vi "CapacityTest.vi"() -> ()   [LabVIEW 2020]
uses:
  <instrlib>/NH Research Regenerative Test Series/Public/Configure/Output Safety.ctl
  <vilib>/DAQmx/read.llb/DAQmx Read (Analog 1D DBL NChan 1Samp).vi
  <vilib>/DAQmx/miscellaneous.llb/DAQmx Fill In Error Info.vi
  <instrlib>/NH Research Regenerative Test Series/Public/Data/Read (Ave Current).vi
  <instrlib>/NH Research Regenerative Test Series/Public/Data/Low Level/Fetch (Ave Voltage).vi
  <instrlib>/NH Research Regenerative Test Series/Public/Data/Low Level/Fetch (Ave True Power).vi
  <instrlib>/NH Research Regenerative Test Series/NH Research Regenerative Test Series.lvlib
panel:
  out "ChamberTemp":dbl
  out "BatteryTemp":dbl
  out "Task error out":errorcluster
  out "String":string
  in  "Output Safety":T1
  out "Filename Out":path
  in  "DAQmx Task Name":refnum<k21>
  out "Voltage Compare":dbl
  in  "Path":path
  in  "Discharge Voltage Setpoint (0 V)":dbl
  out "Ave Current (A)":dbl
  out "Ave Voltage (V)":dbl
  out "Ave True Power (W)":dbl
  out "Status Byte Register":T2
  in  "Logical Instrument Number":u32=1
  in  "Current Setpoint (0 A)":dbl format="%#.6g"
  in  "Voltage Setpoint (0 V)":dbl format="%#.6g"
  in  "Battery Detect Voltage (0V)":dbl format="%#.6g"
  in  "VISA resource name":refnum<visa-resource-name>
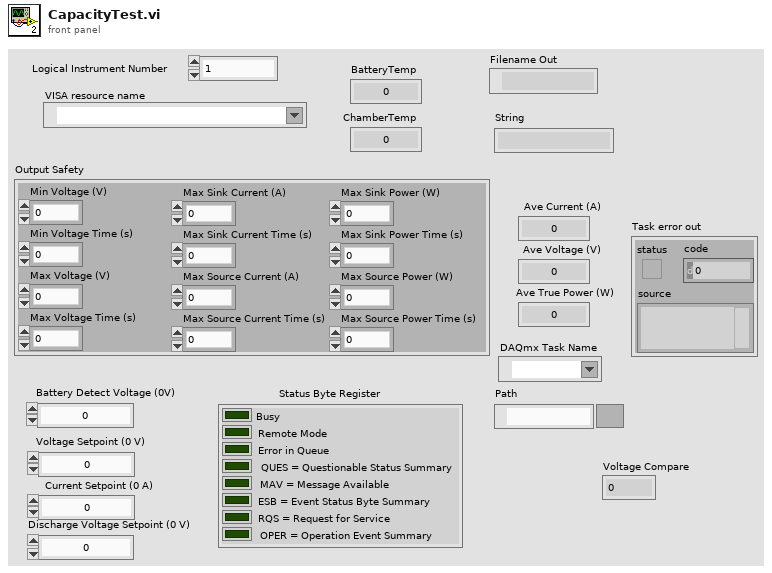
[diagram p1: front panel]
types:
  T1 = typedef "NH Research Regenerative Test Series.lvlib/Output Safety.ctl" = cluster{"Min Voltage (V)":dbl, "Min Voltage Time (s)":dbl, "Max Voltage (V)":dbl, "Max Voltage Time (s)":dbl, "Max Sink Current (A)":dbl, "Max Sink Current Time (s)":dbl, "Max Source Current (A)":dbl, "Max Source Current Time (s)":dbl, "Max Sink Power (W)":dbl, "Max Sink Power Time (s)":dbl, "Max Source Power (W)":dbl, "Max Source Power Time (s)":dbl}
  T2 = cluster{"Busy":bool, "Remote Mode":bool, "Error in Queue":bool, "QUES = Questionable Status Summary":bool, "MAV = Message Available":bool, "ESB = Event Status Byte Summary":bool, "RQS = Request for Service":bool, "OPER = Operation Event Summary":bool}
  T3 = cluster{"data[0]":dbl, "data[1]":dbl, "data[2]":dbl, "data[3]":dbl, "data[4]":dbl, "data[5]":dbl, "data[6]":dbl, "data[7]":dbl, "data[8]":dbl}
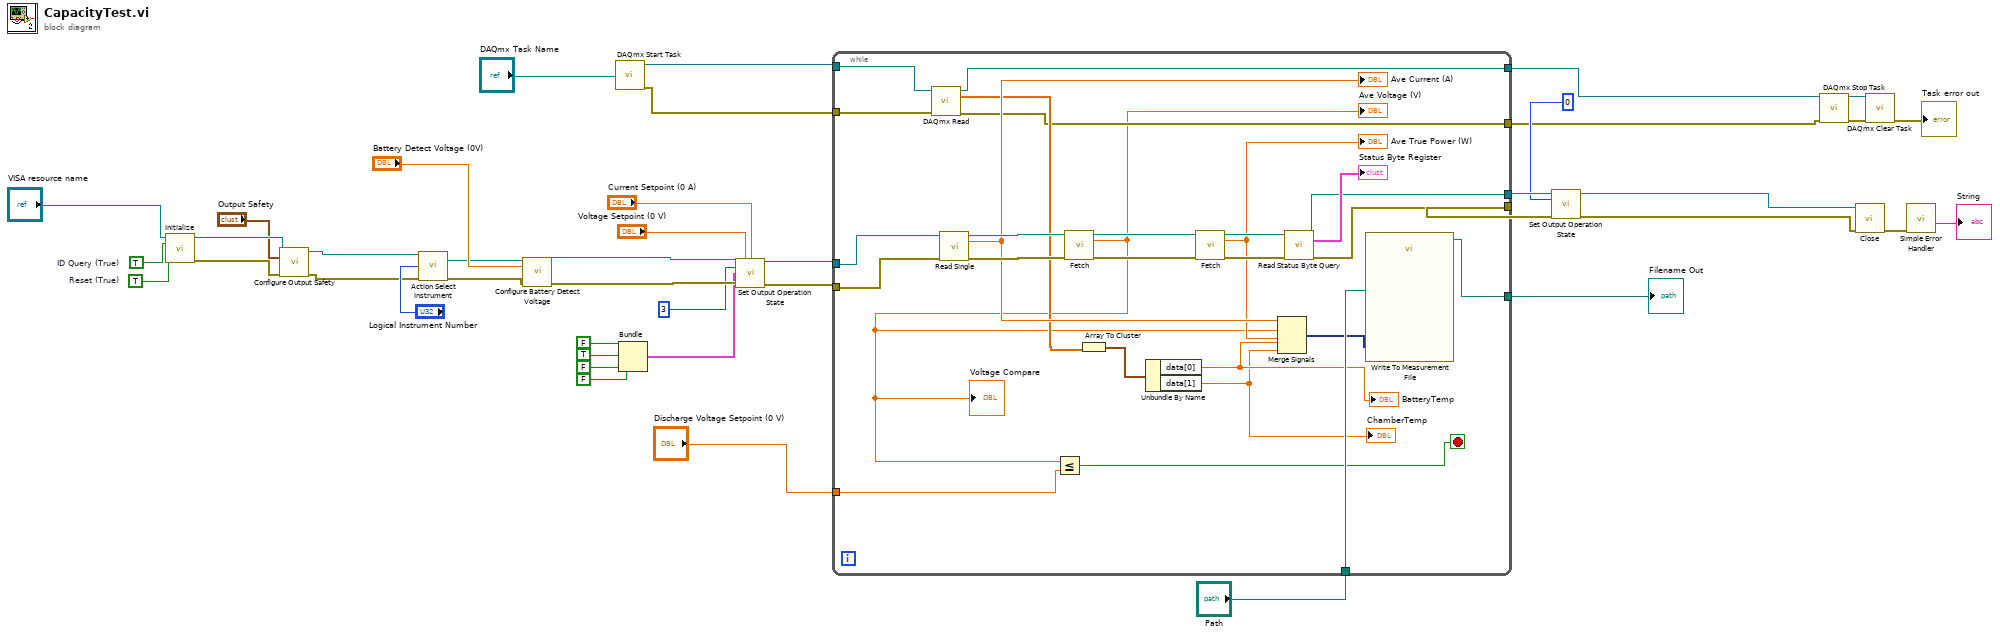
[diagram p0: block diagram]
diagram:
  w20 = TRUE  # ID Query (True)
  w19 = TRUE  # Reset (True)
  n1 = call <vilib>:"Initialize.vi"("VISA resource name"="VISA resource name", "ID Query (True)"=w20, "Reset (True)"=w19) -> ("VISA resource name out"=w18:refnum<visa-resource-name>, "error out"=w17:errorcluster)  [unwired: 11 in]
  n2 = call <vilib>:"Configure Output Safety.vi"("VISA resource name"=w18, "Output Safety"="Output Safety", "error in (no error)"=w17) -> ("VISA resource name out"=w14:refnum<visa-resource-name>, "error out"=w1:errorcluster)  [unwired: 11 in]
  n3 = call <instrlib>:"Action Select Instrument.vi"("VISA resource name"=w14, "Logical Instrument Number"="Logical Instrument Number", "error in (no error)"=w1) -> ("VISA resource name out"=w39:refnum<visa-resource-name>, "error out"=w38:errorcluster)  [unwired: 11 in]
  n4 = call <vilib>:"Configure Battery Detect Voltage.vi"("VISA resource name"=w39, "Battery Detect Voltage (0V)"="Battery Detect Voltage (0V)", "error in (no error)"=w38) -> ("VISA resource name out"=w37:refnum<visa-resource-name>, "error out"=w36:errorcluster)  [unwired: 11 in]
  n5 = call <vilib>:"DAQmx Start Task.vi"("task/channels in"="DAQmx Task Name") -> ("task out"=w12:refnum<k21>, "error out"=w2:errorcluster)  [unwired: 13 in]
  n6 = Bundle(FALSE, TRUE, FALSE, FALSE) -> (w24:cluster{bool, bool, bool, bool})  [unwired: 1 in]
  n7 = call <vilib>:"Set Output Operation State.vi"("VISA resource name"=w37, "Voltage Setpoint (0 V)"="Voltage Setpoint (0 V)", "Current Setpoint (0 A)"="Current Setpoint (0 A)", "Mode (0: Off)"=3, "Enable"=w24, "error in (no error)"=w36) -> ("VISA resource name out"=w32:refnum<visa-resource-name>, "error out"=w31:errorcluster)  [unwired: 8 in]
  n8 = while {
    tunnel: w32 -> [w63]
    tunnel: w31 -> [w62]
    tunnel: [w60] -> w35
    tunnel: [w59] -> w34
    tunnel: "Discharge Voltage Setpoint (0 V)" -> [w46]
    tunnel: "Path" -> [w56]
    tunnel: w12 -> [w55]
    tunnel: [w51] -> w4
    tunnel: [w50] -> w3
    tunnel: w2 -> [w49]
    tunnel: [w48] -> w21
    stop <- w47 stop-if-true
    n9 = call-poly <vilib>:"DAQmx Read.vi"("task/channels in"=w55, "error in"=w49) -> ("task out"=w51:refnum<k21>, "data"=w54:dbl[], "error out"=w50:errorcluster)  [unwired: 11 in]
    n10 = call-poly <instrlib>:"Read Single.vi"("VISA resource name"=w63, "error in (no error)"=w62) -> ("VISA resource name out"=w68:refnum<visa-resource-name>, "Ave Current (A)"=w58:dbl, "error out"=w69:errorcluster)  [unwired: 11 in]
    "Ave Current (A)" <- w58
    n11 = call-poly <instrlib>:"Fetch.vi"("VISA resource name"=w68, "error in (no error)"=w69) -> ("VISA resource name out"=w67:refnum<visa-resource-name>, "Ave Voltage (V)"=w45:dbl, "error out"=w66:errorcluster)  [unwired: 11 in]
    "Ave Voltage (V)" <- w45
    "Voltage Compare" <- w45
    n12 = Less Or Equal?(x=w45, y=w46) -> (x <= y?=w47:bool)
    n13 = Array To Cluster(array=w54) -> (cluster=w53:T3)
    n14 = Unbundle By Name(w53) -> ("data[0]"=w44:dbl, "data[1]"=w43:dbl)
    "BatteryTemp" <- w44
    "ChamberTemp" <- w43
    n15 = call-poly <instrlib>:"Fetch.vi"("VISA resource name"=w67, "error in (no error)"=w66) -> ("VISA resource name out"=w65:refnum<visa-resource-name>, "Ave True Power (W)"=w57:dbl, "error out"=w64:errorcluster)  [unwired: 11 in]
    "Ave True Power (W)" <- w57
    n16 = Merge Signals "Merge Signals"(w58, w45, w57, w44, w43) -> (w52:dynamicdata)
    n17 = call <instrlib>:"Read Status Byte Query.vi"("VISA resource name"=w65, "error in (no error)"=w64) -> ("VISA resource name out"=w60:refnum<visa-resource-name>, "Status Byte Register"=→"Status Byte Register":T2, "error out"=w59:errorcluster)  [unwired: 11 in]
    n18 = call "Write To Measurement File"("Signals"=w52, "Filename"=w56) -> ("Filename Out"=w48:path)  [unwired: 15 in, 2 out]
  }
  "Filename Out" <- w21
  n19 = call <vilib>:"Set Output Operation State.vi"("VISA resource name"=w35, "Mode (0: Off)"=0, "error in (no error)"=w34) -> ("VISA resource name out"=w6:refnum<visa-resource-name>, "error out"=w5:errorcluster)  [unwired: 11 in]
  n20 = call <vilib>:"DAQmx Stop Task.vi"("task/channels in"=w4, "error in"=w3) -> ("task out"=w10:refnum<k21>, "error out"=w9:errorcluster)  [unwired: 12 in]
  n21 = call <instrlib>:"Close.vi"("VISA resource name"=w6, "error in (no error)"=w5) -> ("error out"=w7:errorcluster)  [unwired: 13 in]
  n22 = call <vilib>:"DAQmx Clear Task.vi"("task in"=w10, "error in"=w9) -> ("error out"=→"Task error out":errorcluster)  [unwired: 13 in]
  n23 = call <vilib>:"Simple Error Handler.vi"("error in (no error)"=w7) -> ("source out"=→"String":string)  [unwired: 4 in, 4 out]
